vi "CRC.vi"(1 "Input String":string) -> (0 "String w/ CRC":string)   [LabVIEW 2015]
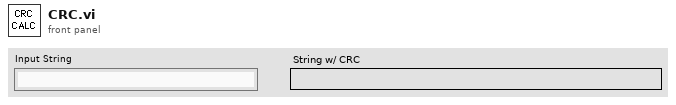
[diagram p1: front panel]
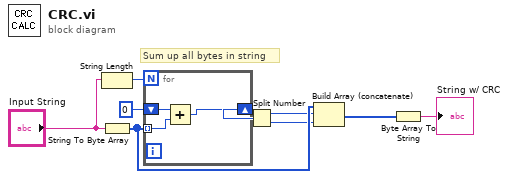
[diagram p0: block diagram]
diagram:
  # "Sum up all bytes in string"
  n1 = String Length(string="Input String") -> (length=w9:i32)
  n2 = String To Byte Array(string="Input String") -> (unsigned byte array=w5:u8[])
  n3 = for {
    N: w9 -> [_]
    tunnel: w5 -> [w12] mode=indexing
    shift-right: [w11] -> w6
    shift-left: u16 0 -> [w10]
    n4 = Add(x=w10, y=w12) -> (x+y=w11:u16)
  }
  n5 = Split Number(x=w6) -> (hi(x)=w4:u8, lo(x)=w3:u8)
  n6 = Build Array (concatenate)(w5, w4, w3) -> (w2:u8[])
  n7 = Byte Array To String(unsigned byte array=w2) -> (string=→"String w/ CRC":string)
